vi "Calculator.vi"(8 "error in (no error)":errorcluster, 9 "Input 2":i32, 10 "Input 1":i32, 11 "Calculator in":refnum<class "Calculator.lvclass">) -> (0 "error out":errorcluster, 2 "Output":i32, 3 "Calculator out":refnum<class "Calculator.lvclass">)   [LabVIEW 2020, in "Calculator.lvclass"]
uses:
  LabVIEW Data/Calculator/Calculator.lvclass
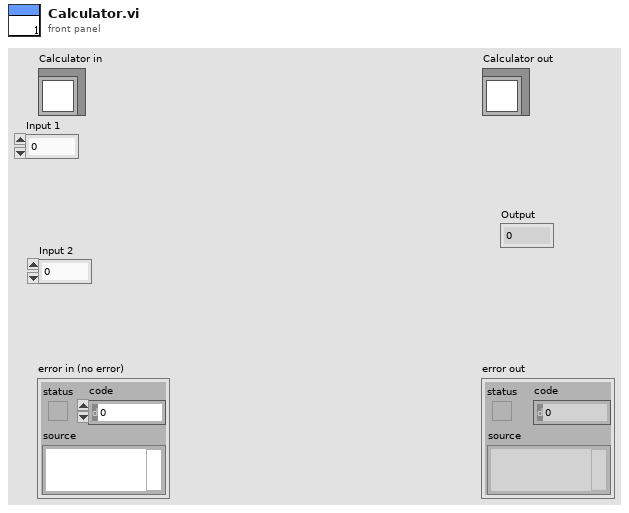
[diagram p1: front panel]
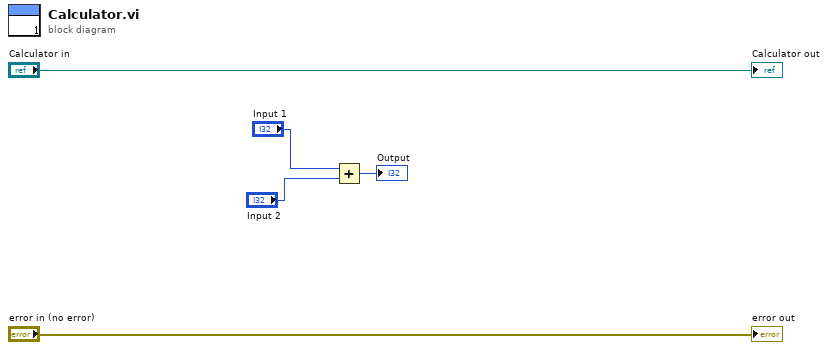
[diagram p0: block diagram]
diagram:
  n1 = Add(x="Input 1", y="Input 2") -> (x+y=→"Output":i32)
  "error out" <- "error in (no error)"
  "Calculator out" <- "Calculator in"
